vi "ImplModelFollow_New_Plant.vi"(9 "PlantRef":T1, 11 "Plant":T1) -> (0 "Error":bool, 3 "IMPLICIT_MODEL_FOLLOWER":T3)   [LabVIEW 2019, in "Trajectory_Library.lvlib"]
doc: "Create implicit model follower\n\nInputs:\n - A < states, states > -- Continuous system matrix of the plant being controlled.\n - B < states, inputs > -- Continuous input matrix of the plant being controlled.\n - A_Ref < states, states > -- Continuous system matrix whose dymanics should be followed.\n - B_Ref < states, inputs > -- Continuous input matrix x whose dymanics should be followed.\n\nOutputs:\n - Error -- If TRUE, an error occured."
uses:
  Trajectory_Library.lvlib
  <vilib>/Analysis/Matrix/Datatypes/RealMatrix.ctl
  <vilib>/Analysis/Matrix/NI_Matrix.lvlib
  TypeDef/IMPLICIT_MODEL_FOLLOWER.ctl
  TypeDef/LINEAR_SYSTEM.ctl
panel:
  # "<States,States>"
  # "<States,Inputs>"
  # "<Outputs,States>"
  # "<Outputs,Inputs>"
  # "<States,States>"
  # "<States,Inputs>"
  # "<Outputs,States>"
  # "<Outputs,Inputs>"
  # "<States,States>"
  # "<States,Inputs>"
  # "<Inputs,1>"
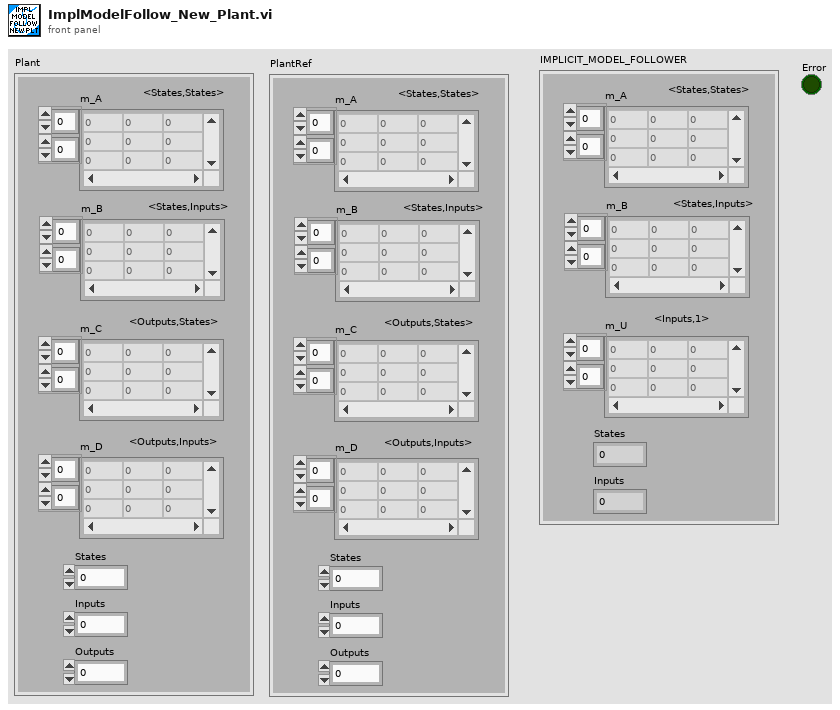
[diagram p1: front panel]
types:
  T1 = typedef "Trajectory_Library.lvlib/LINEAR_SYSTEM.ctl" = cluster{"m_A":T2, "m_B":T2, "m_C":T2, "m_D":T2, "States":i32, "Inputs":i32, "Outputs":i32}
  T2 = typedef "NI_Matrix.lvlib/RealMatrix.ctl" = dbl[][]
  T3 = typedef "Trajectory_Library.lvlib/IMPLICIT_MODEL_FOLLOWER.ctl" = cluster{"m_A":T2, "m_B":T2, "m_U":T2, "States":i32, "Inputs":i32}
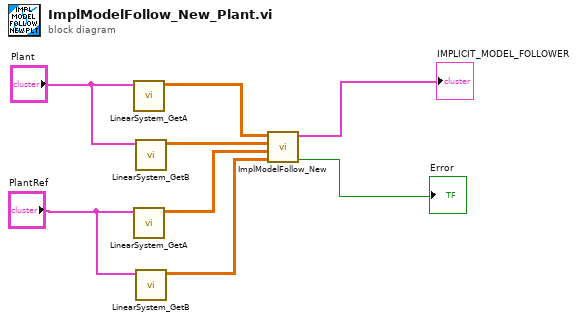
[diagram p0: block diagram]
diagram:
  n1 = call "LinearSystem_GetA.vi"("Linearsystem"="Plant") -> ("A"=w6:T2)  [unwired: 10 in]
  n2 = call "LinearSystem_GetA.vi"("Linearsystem"="PlantRef") -> ("A"=w4:T2)  [unwired: 10 in]
  n3 = call "LinearSystem_GetB.vi"("Linearsystem"="Plant") -> ("B"=w5:T2)  [unwired: 10 in]
  n4 = call "LinearSystem_GetB.vi"("Linearsystem"="PlantRef") -> ("B"=w3:T2)  [unwired: 10 in]
  n5 = call "ImplModelFollow_New.vi"("B_Ref"=w3, "A_Ref"=w4, "B"=w5, "A"=w6) -> ("Error"=→"Error":bool, "IMPLICIT_MODEL_FOLLOWER"=→"IMPLICIT_MODEL_FOLLOWER":T3)  [unwired: 6 in]
